vi "StageStatus (SubVI).vi"(7 "Aerotech reference IN":refnum<k24>, 8 "error in (no error)":errorcluster, 11 "Axes Names":string[](array[string])) -> (0 "error out":errorcluster, 1 "Z Position Feedback":dbl, 2 "Y Position Feedback":dbl, 3 "X Position Feedback":dbl, 4 "Current stage position":T2, 5 "Aerotech reference OUT":refnum<k24>, 6 "Axes' current status display":T1[](array[typedef]))   [LabVIEW 2017]
doc: "Returns the Aerotech XYZ stage's current position per axis, or as a cluster with elements X position, Y position, and Z position. The units reflect those of the XYZ stage, so all the lengths are in mm. \n\nBuilt on top of the Aerotech .NET Libraries."
uses:
  AerotechLibraries/Status/AxisDiagPacket.ctl
panel:
  # "SubVI to retrieve the current position of the XYZ stage"
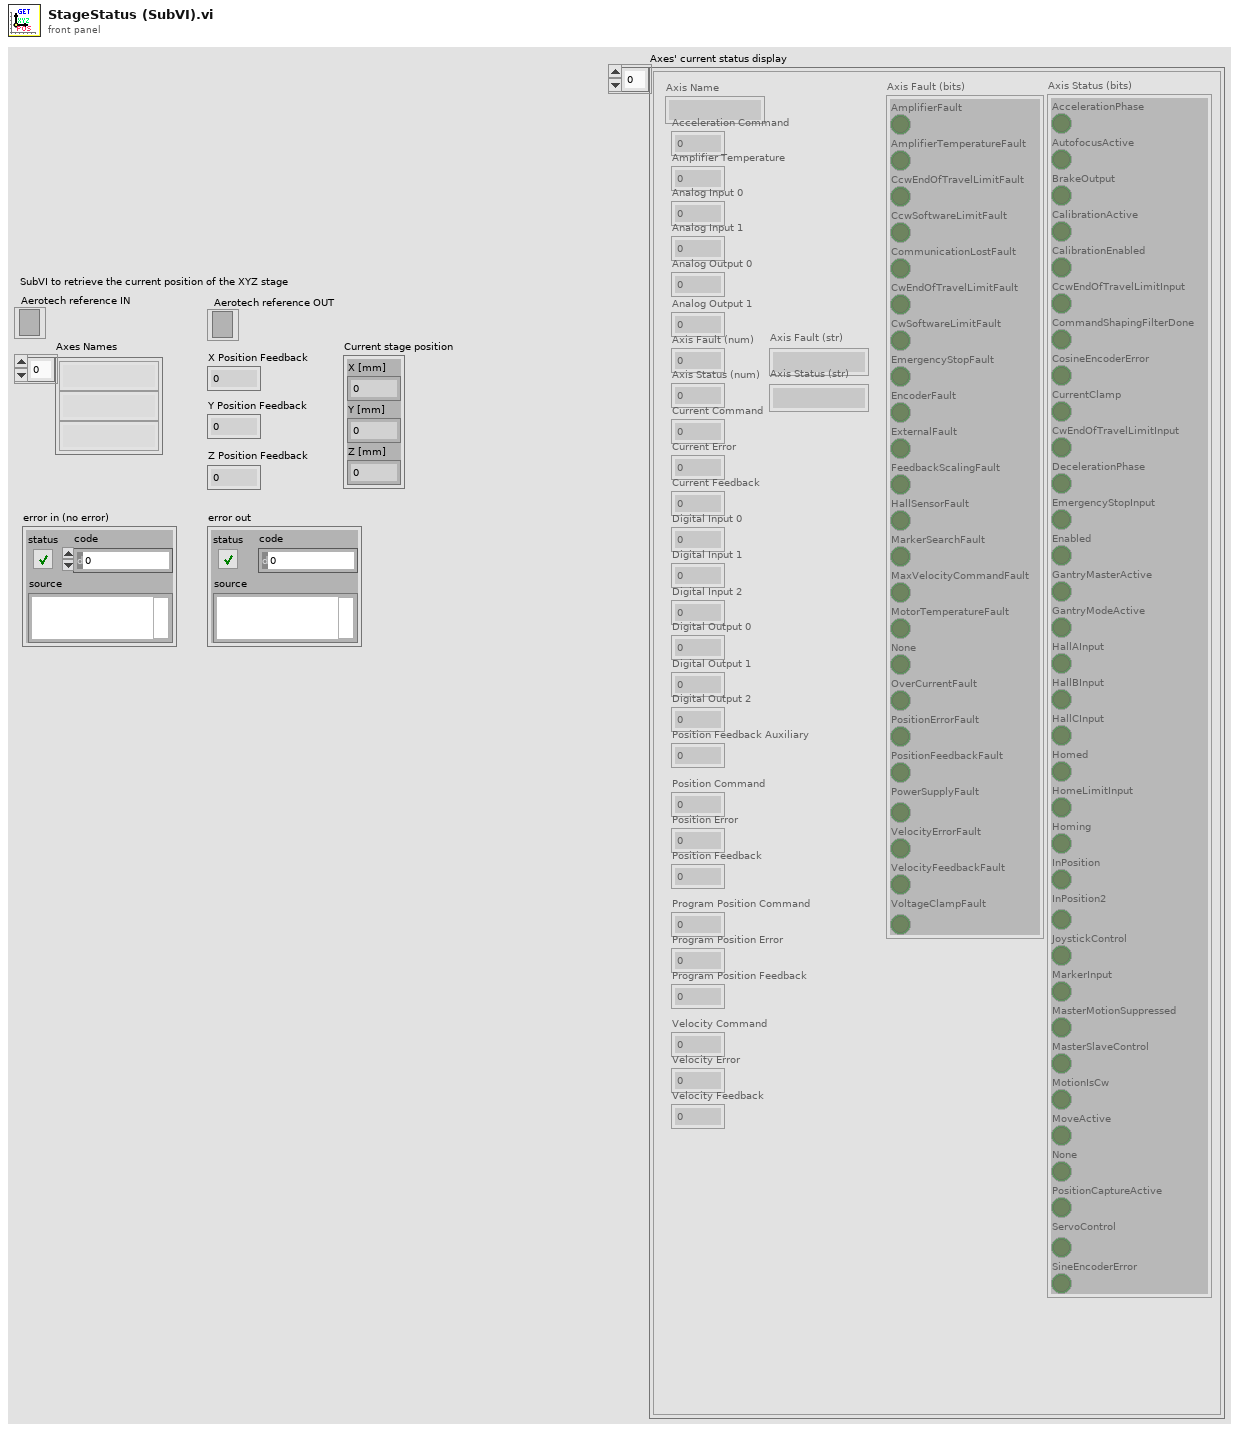
[diagram p1: front panel]
types:
  T1 = typedef "AxisDiagPacket.ctl" = cluster{"Axis Name":string, "Acceleration Command":dbl, "Amplifier Temperature":sgl, "Analog Input 0":dbl, "Analog Input 1":dbl, "Analog Output 0":dbl, "Analog Output 1":dbl, "Axis Fault (num)":i32, "Axis Fault (str)":string, "Axis Fault (bits)":cluster{"AmplifierFault":bool, "AmplifierTemperatureFault":bool, "CcwEndOfTravelLimitFault":bool, "CcwSoftwareLimitFault":bool, "CommunicationLostFault":bool, "CwEndOfTravelLimitFault":bool, "CwSoftwareLimitFault":bool, "EmergencyStopFault":bool, "EncoderFault":bool, "ExternalFault":bool, "FeedbackScalingFault":bool, "HallSensorFault":bool, "MarkerSearchFault":bool, "MaxVelocityCommandFault":bool, "MotorTemperatureFault":bool, "None":bool, "OverCurrentFault":bool, "PositionErrorFault":bool, "PositionFeedbackFault":bool, "PowerSupplyFault":bool, "VelocityErrorFault":bool, "VelocityFeedbackFault":bool, "VoltageClampFault":bool}, "Axis Status (num)":i32, "Axis Status (str)":string, "Axis Status (bits)":cluster{"AccelerationPhase":bool, "AutofocusActive":bool, "BrakeOutput":bool, "CalibrationActive":bool, "CalibrationEnabled":bool, "CcwEndOfTravelLimitInput":bool, "CommandShapingFilterDone":bool, "CosineEncoderError":bool, "CurrentClamp":bool, "CwEndOfTravelLimitInput":bool, "DecelerationPhase":bool, "EmergencyStopInput":bool, "Enabled":bool, "GantryMasterActive":bool, "GantryModeActive":bool, "HallAInput":bool, "HallBInput":bool, "HallCInput":bool, "Homed":bool, "HomeLimitInput":bool, "Homing":bool, "InPosition":bool, "InPosition2":bool, "JoystickControl":bool, "MarkerInput":bool, "MasterMotionSuppressed":bool, "MasterSlaveControl":bool, "MotionIsCw":bool, "MoveActive":bool, "None":bool, "PositionCaptureActive":bool, "ServoControl":bool, "SineEncoderError":bool}, "Current Command":sgl, "Current Error":sgl, "Current Feedback":sgl, "Digital Input 0":i32, "Digital Input 1":i32, "Digital Input 2":i32, "Digital Output 0":i32, "Digital Output 1":i32, "Digital Output 2":i32, "Position Feedback Auxiliary":dbl, "Position Command":dbl, "Position Error":dbl, "Position Feedback":dbl, "Program Position Command":dbl, "Program Position Error":dbl, "Program Position Feedback":dbl, "Velocity Command":dbl, "Velocity Error":dbl, "Velocity Feedback":dbl}
  T2 = cluster{"X [mm]":dbl, "Y [mm]":dbl, "Z [mm]":dbl}
  T3 = typedef "ControllerDiagPacket.ctl" = cluster{"Count":i32, "Packet Time":i64, "Axes":T1[], "error":errorcluster}
  T4 = cluster{"Axes Names[0]":string, "Axes Names[1]":string, "Axes Names[2]":string, "Axes Names[3]":string, "Axes Names[4]":string, "Axes Names[5]":string, "Axes Names[6]":string, "Axes Names[7]":string, "Axes Names[8]":string}
  T5 = cluster{"Program Position Feedback":dbl, "Program Position Feedback":dbl, "Program Position Feedback":dbl}
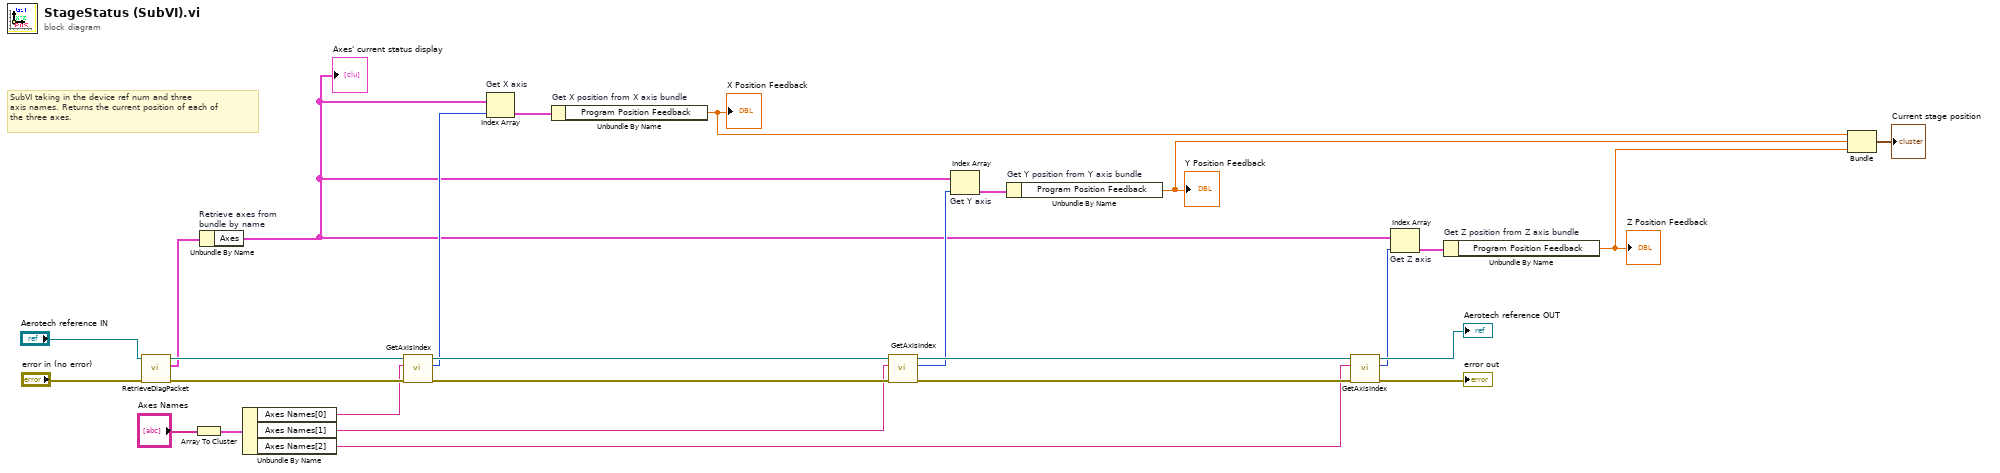
[diagram p0: block diagram]
diagram:
  # "SubVI taking in the device ref num and three\naxis names. Returns the current position of each of\nthe three axes."
  n1 = call "RetrieveDiagPacket.vi"("error in (no error)"="error in (no error)", "Controller In"="Aerotech reference IN") -> ("error out"=w18:errorcluster, "ControllerDiagPacket"=w15:T3, "Controller Out"=w20:refnum<k24>)  [unwired: 7 in]
  n2 = Array To Cluster(array="Axes Names") -> (cluster=w16:T4)
  n3 = Unbundle By Name "Retrieve axes from bundle by name"(w15) -> ("Axes"=w8:T1[])
  "Axes' current status display" <- w8
  n4 = Unbundle By Name(w16) -> ("Axes Names[0]"=w7:string, "Axes Names[1]"=w6:string, "Axes Names[2]"=w5:string)
  n5 = call "GetAxisIndex.vi"("error in (no error)"=w18, "axis name"=w7, "controller in"=w20) -> ("error out"=w19:errorcluster, "axis index"=w14:i32, "controller out"=w21:refnum<k24>)  [unwired: 6 in]
  n6 = Index Array "Get X axis"(array=w8, index=w14) -> (element=w13:T1)
  n7 = Unbundle By Name "Get X position from X axis bundle"(w13) -> ("Program Position Feedback"=w4:dbl)
  "X Position Feedback" <- w4
  n8 = call "GetAxisIndex.vi"("error in (no error)"=w19, "axis name"=w6, "controller in"=w21) -> ("error out"=w24:errorcluster, "axis index"=w12:i32, "controller out"=w26:refnum<k24>)  [unwired: 6 in]
  n9 = Index Array "Get Y axis"(array=w8, index=w12) -> (element=w11:T1)
  n10 = Unbundle By Name "Get Y position from Y axis bundle"(w11) -> ("Program Position Feedback"=w3:dbl)
  "Y Position Feedback" <- w3
  n11 = call "GetAxisIndex.vi"("error in (no error)"=w24, "axis name"=w5, "controller in"=w26) -> ("error out"=→"error out":errorcluster, "axis index"=w9:i32, "controller out"=→"Aerotech reference OUT":refnum<k24>)  [unwired: 6 in]
  n12 = Index Array "Get Z axis"(array=w8, index=w9) -> (element=w10:T1)
  n13 = Unbundle By Name "Get Z position from Z axis bundle"(w10) -> ("Program Position Feedback"=w2:dbl)
  "Z Position Feedback" <- w2
  n14 = Bundle("Program Position Feedback"=w4, "Program Position Feedback"=w3, "Program Position Feedback"=w2) -> (→"Current stage position":T5)  [unwired: 1 in]
